vi "Setup.vi"(8 "error in":errorcluster, 11 "Sensormetrix COM port":refnum<visa-resource-name>) -> (0 "error out":errorcluster, 3 "Modbus master out":refnum<class "Modbus Master.lvclass">)   [LabVIEW 2014, in "T3110 & T2114.lvlib"]
uses:
  T3110 & T2114.lvlib
  <vilib>/NI/Modbus Library/API/Master/Modbus Master.lvclass
  <vilib>/NI/Modbus Library/API/Wrapper/Create Serial Master.vi
  <vilib>/NI/Modbus Library/API/Wrapper/API Main.lvlib
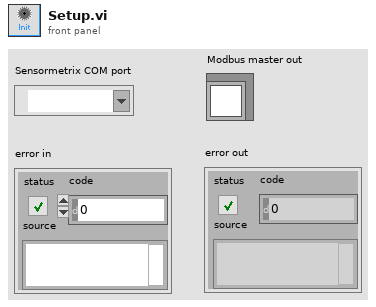
[diagram p1: front panel]
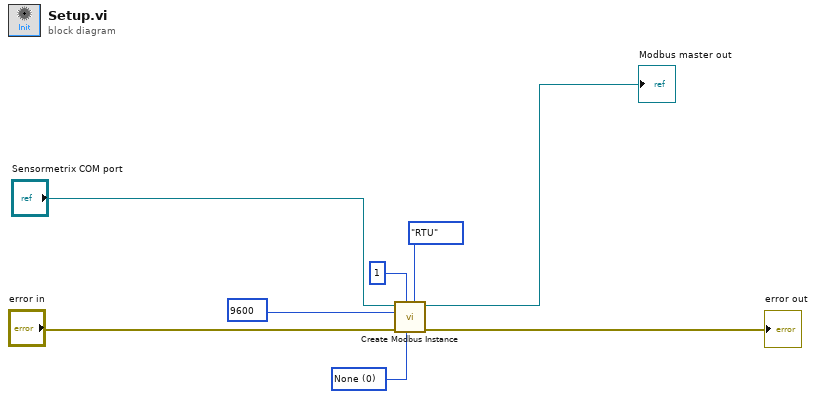
[diagram p0: block diagram]
diagram:
  w3 = u16 0 items=["None", "Odd", "Even", "Mark", "Space"] ("parity (even)")
  n1 = call-poly <vilib>:"Create Modbus Instance.vi"("serial type"=enum16{"RTU", "ASCII"}."RTU", "parity (even)"=w3, "unit ID"=u8 1, "error in"="error in", "baud rate"=u32 9600, "VISA resource name"="Sensormetrix COM port") -> ("error out"=→"error out":errorcluster, "serial master instance"=→"Modbus master out":refnum<class "Modbus Master.lvclass">)  [unwired: 4 in]
